vi "Run Tx - Echo Transmit.vi"(6 "Transmitted?":bool, 7 "Echo Resources in":T1, 8 "error in (no error)":errorcluster, 11 "Transmit Echo":T3) -> (0 "error out":errorcluster, 5 "Echo Resources out":T1)   [LabVIEW 2021, in "UDP-Custom-Device Engine.lvlib"]
uses:
  UDP-Custom-Device Engine.lvlib
  <vilib>/NI/NIVS Inline Async API/_Data Access Engine/Data Access Engine/Types/Write.DVR.ctl
  <vilib>/NI/NIVS Inline Async API/_Data Access Engine/Access Type Classes/Write/Write.lvclass
  Types/Engine - Tx Echo Resources.ctl
  Shared/Types/Shared - Transmit Echo Options.ctl
  <vilib>/NI/NIVS Inline Async API/_Data Access Engine/Access Type Classes/Write/Write.lvclass/Write.ctl
  <vilib>/NI/NIVS Inline Async API/_Data Access Engine/Data Access Engine/Methods/Write.Data.vi
  <vilib>/NI/NIVS Inline Async API/_Data Access Engine/Access Type Classes/Write/Write.ProcessData.vi
  <vilib>/NI/NIVS Inline Async API/_Data Access Engine/Access Type Classes/Write/Write.Buffer.vi
  <vilib>/NI/NIVS Inline Async API/_Data Access Engine/Access Type Classes/Write/Write.Commit.vi
  <vilib>/NI/NIVS Inline Async API/_Data Access Engine/Data Access Engine/Data Access Engine.lvclass
  Shared/UDP-Custom-Device Shared.lvlib
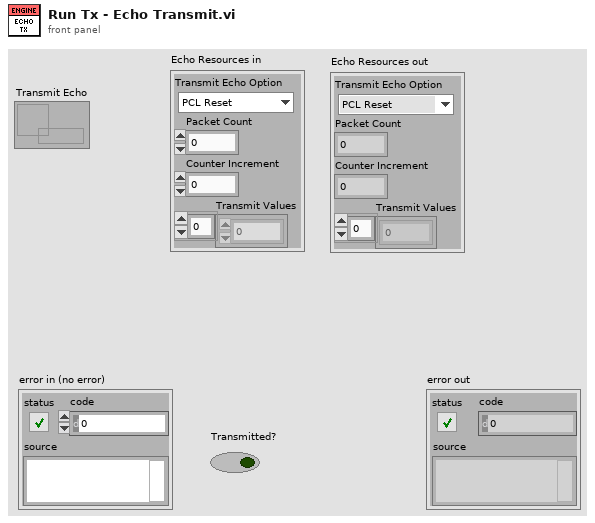
[diagram p1: front panel]
types:
  T1 = typedef "UDP-Custom-Device Engine.lvlib/Engine - Tx Echo Resources.ctl" = cluster{"Transmit Echo Option":T2, "Packet Count":dbl, "Counter Increment":dbl, "Transmit Values":dbl[]}
  T2 = typedef "UDP-Custom-Device Shared.lvlib/Shared - Transmit Echo Options.ctl" = enum16{"PCL Reset", "Counter", "Mirror"}
  T3 = typedef "Data Access Engine.lvlib/Data Access Engine.lvclass/Write.DVR.ctl" = refnum<data-value>
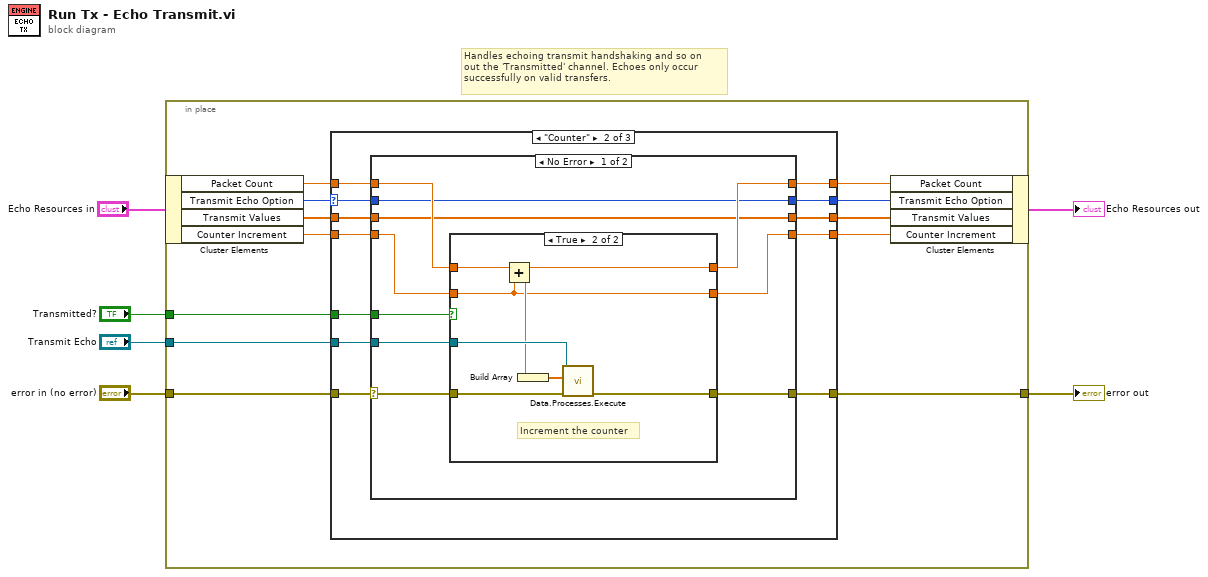
[diagram p0: block diagram]
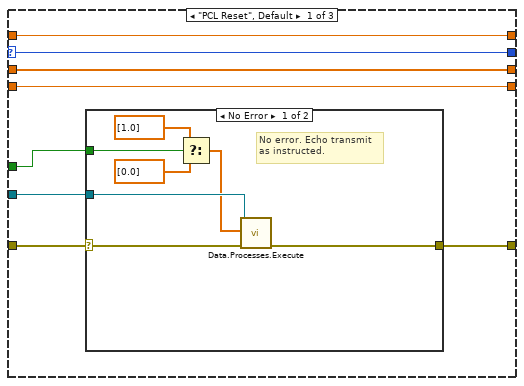
[diagram p2: hidden frame]
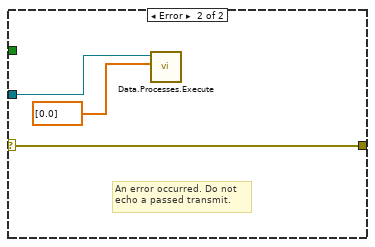
[diagram p3: hidden frame]
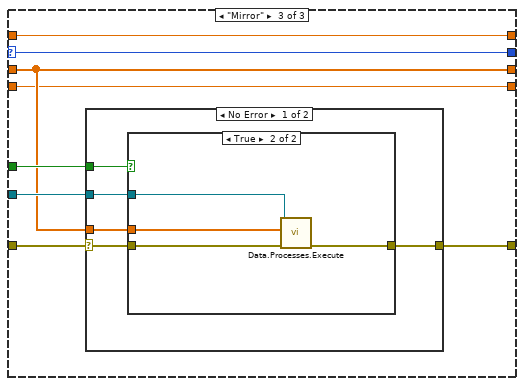
[diagram p6: hidden frame]
diagram:
  # "Handles echoing transmit handshaking and so on\nout the 'Transmitted' channel. Echoes only occur\nsuccessfully on valid transfers."
  n1 = in-place {
    in-place-border: "error in (no error)" -> [w18]
    in-place-border: "Transmit Echo" -> [w17]
    in-place-border: "Transmitted?" -> [w16]
    in-place-border: [w15] -> w3
    n2 = in-place-cluster #1("Echo Resources in") -> ("Packet Count"=w13:dbl, "Transmit Echo Option"=w14:T2, "Transmit Values"=w10:dbl[], "Counter Increment"=w8:dbl)
    n3 = case shown="\"Counter\"" w14 {
      selector: w14 -> [w21 w42 w76]
      tunnel: w18 -> [w26 w48 w81]
      tunnel: w17 -> [w25 w47 w80]
      tunnel: w16 -> [w24 w46 w79]
      tunnel: [w23 w45 w78] -> w15
      tunnel: w13 -> [w20 w44 w75]
      tunnel: [w20 w43 w75] -> w12
      tunnel: [w21 w41 w76] -> w11
      tunnel: w10 -> [w22 w40 w77]
      tunnel: [w22 w39 w77] -> w9
      tunnel: w8 -> [w19 w38 w74]
      tunnel: [w19 w37 w74] -> w7
      frame "PCL Reset", Default {
        n4 = case shown="No Error" w26 {
          selector: w26 -> [w33 w34]
          tunnel: w25 -> [w31 w36]
          tunnel: w24 -> [w30 _]
          tunnel: [w32 w34] -> w23
          frame No Error {
            # "No error. Echo transmit\nas instructed."
            n5 = Select(t=dbl[] [1.0] ("Values"), s=w30, f=dbl[] [0.0] ("Values")) -> (s? t:f=w27:dbl[])
            n6 = call-poly <vilib>:"Data.Processes.Execute.vi"("error in (no error)"=w33, "Values"=w27, "Ref"=w31) -> ("error out"=w32:errorcluster)  [unwired: 8 in]
          }
          frame Error {
            # "An error occurred. Do not\necho a passed transmit."
            n7 = call-poly <vilib>:"Data.Processes.Execute.vi"("Values"=dbl[] [0.0], "Ref"=w36) -> ()  [unwired: 9 in, 1 out]
          }
        }
      }
      frame "Counter" {
        n8 = case shown="No Error" w48 {
          selector: w48 -> [w58 w72]
          tunnel: w47 -> [w56 _]
          tunnel: w46 -> [w54 _]
          tunnel: [w57 w72] -> w45
          tunnel: w44 -> [w55 w73]
          tunnel: [w53 w73] -> w43
          tunnel: w42 -> [w51 w71]
          tunnel: [w51 w71] -> w41
          tunnel: w40 -> [w52 w70]
          tunnel: [w52 w70] -> w39
          tunnel: w38 -> [w50 w69]
          tunnel: [w49 w69] -> w37
          frame No Error {
            n9 = case shown="True" w54 {
              tunnel: w58 -> [w60 w68]
              tunnel: [w60 w67] -> w57
              tunnel: w56 -> [_ w66]
              tunnel: w55 -> [w61 w65]
              tunnel: [w61 w63] -> w53
              tunnel: w50 -> [w59 w62]
              tunnel: [w59 w62] -> w49
              frame False {
                # "Do not increment the counter"
              }
              frame True {
                # "Increment the counter"
                n10 = Add(x=w65, y=w62) -> (x+y=w63:dbl)
                n11 = Build Array(w63) -> (w64:dbl[])
                n12 = call-poly <vilib>:"Data.Processes.Execute.vi"("error in (no error)"=w68, "Values"=w64, "Ref"=w66) -> ("error out"=w67:errorcluster)  [unwired: 8 in]
              }
            }
          }
          frame Error {
            # "An error occurred. Do not\nincrement"
          }
        }
      }
      frame "Mirror" {
        n13 = case shown="No Error" w81 {
          selector: w81 -> [w86 w92]
          tunnel: w80 -> [w84 _]
          tunnel: w79 -> [w83 _]
          tunnel: [w85 w92] -> w78
          tunnel: w77 -> [w82 _]
          frame No Error {
            n14 = case shown="True" w83 {
              tunnel: w86 -> [w87 w91]
              tunnel: [w87 w90] -> w85
              tunnel: w84 -> [_ w89]
              tunnel: w82 -> [_ w88]
              frame False {
              }
              frame True {
                n15 = call-poly <vilib>:"Data.Processes.Execute.vi"("error in (no error)"=w91, "Values"=w88, "Ref"=w89) -> ("error out"=w90:errorcluster)  [unwired: 8 in]
              }
            }
          }
          frame Error {
            # "An error occurred. Do not update\nthe mirror."
          }
        }
      }
    }
    n16 = in-place-cluster #1("Packet Count"=w12, "Transmit Echo Option"=w11, "Transmit Values"=w9, "Counter Increment"=w7) -> (→"Echo Resources out":T1)
  }
  "error out" <- w3
